vi "macro_vecBuilder1x1FIll.vi"   [LabVIEW 2019, in "Trajectory_Library.lvlib"]
uses:
  MatBuilder_Create.vi
  Trajectory_Library.lvlib
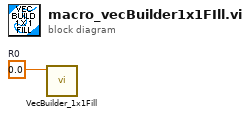
[diagram p0: block diagram]
diagram:
  w1 = 0.0  # R0
  n1 = call "VecBuilder_1x1Fill.vi"("R0_C0"=w1) -> ()  [unwired: 10 in, 1 out]
